vi "Initalize SR830(SubVI).vi"(0 "簇":T1={"initialize"=enum."SR830", "6221"={"6221 Resource"="GPIB0::24::INSTR", "Delta status"=FALSE, "电流|RMS(A)"=0.0}, "SR830+6221"={"source"=0, "Current(A)"=0.0, "阻抗(Ohm)"=0.0, "SR830 1"=FALSE, "SR830 2"=FALSE, "SR830 3"=FALSE, "SR830 4"=FALSE, "VISA 1"="", "VISA 2"="", "VISA 3"="", "VISA 4"="", "Reserve 1"=0, "Reserve 2"=-1, "Reserve 3"=-1, "Reserve 4"=-1, "Sensitivity 1"=-1, "Sensitivity 2"=0, "Sensitivity 3"=-1, "Sensitivity 4"=-1, "量程入 1"=0, "量程入 2"=0, "量程入 3"=0, "量程入 4"=0}, "2400"={"2400"=FALSE, "VISA"="", "Output Level (0)"=1e-05, "Compliance  Level (0.1)"=10.0}, "ch"={"ch"=[], "current"=[], "change?"=[], "holding current\nwhen change ch?"=FALSE}, "Instrument"={"325 Resource "="GPIB0::13::INSTR", "Input (0:A) 325"=0, "Heater Output (1:1) 325"=1, "340 Resource"="GPIB0::14::INSTR", "Input (0:A) 340"=0, "Loop (0: 1)"=0, "Input (0:B) 340"=1, "Loop (1: 1)"=0, "340 Status"=refnum, "Instrument Type"=enum."PPMS-Rotate", "quantum design"=refnum, "semaphore 325"=refnum, "TCP master instance"=refnum, "M24C Resource"="GPIB0::24::INSTR", "4G supply"="GPIB0::24::INSTR", "Temp Status 24C"=refnum, "Temp"=refnum, "9T信号"=refnum, "limit"={"Field limit"=0.0, "Field rate limit"=0.0, "Temp limit"=0.0, "Temp low limit"=0.0, "Temp rate limit "=0.0}, "4g supply status"=refnum, "vi路径"="", "in-plane"="", "out-plane"="", "in-plane signal"=FALSE, "out-plane signal"=FALSE, "in plane 信号"=refnum, "pzt volt"=refnum, "Aborting"=refnum, "数据文件"=refnum, "warning"=refnum, "750 visa"="", "750 rotate"="", "335 Status 2"=refnum, "335 Resource "="GPIB0::24::INSTR", "Input (0:A) 335"=0, "Input (0:B) 335"=1, "Heater Output (1:1) 335"=1, "semaphore 340"=refnum, "semaphore 335"=refnum, "325 Status"=refnum, "semaphore 750"=refnum, "750 field status"=refnum, "camg 振荡状态"=refnum, "列表框"=refnum, "编辑列表框？"=refnum, "camg Rate"=refnum, "行数"=refnum}, "2614B"={"2614B chA"=FALSE, "2614B chB"=FALSE, "VISA"=""}, "33522b"={"33522b resource name"="GPIB0::16::INSTR", "零电压"=0.0, "最大电压"=148.0, "间隔"=4.0, "最小电压"=-48.0, "PZT Scan?"=FALSE}, "gating type"=enum."2614(daul)", "层数"=0, "行数"=0, "是否处理"=[]} {"Instrument"."Loop (1: 1)" items=["1"=1, "2"=2]; "Instrument"."Loop (0: 1)" items=["1"=1, "2"=2]; "Instrument"."Input (0:B) 340" items=["A", "B", "C", "D"]; "Instrument"."Heater Output (1:1) 335" items=["1"=1, "2"=2]; "Instrument"."Input (0:B) 335" items=["A", "B"]; "Instrument"."Input (0:A) 335" items=["A", "B"]; "Instrument"."Heater Output (1:1) 325" items=["1"=1, "2"=2]; "Instrument"."Input (0:A) 325" items=["A", "B"]; "Instrument"."Input (0:A) 340" items=["1"=1, "2"=2]; "SR830+6221"."Sensitivity 4" items=["Auto Gain"=-1, "2 nV/fA"=0, "5 nV/fA"=1, "10 nV/fA"=2, "20 nV/fA"=3, "50 nV/fA"=4, "100 nV/fA"=5, "200 nV/fA"=6, "500 nV/fA"=7, "1 uV/pA"=8, "2 uV/pA"=9, "5 uV/pA"=10, "10 uV/pA"=11, "20 uV/pA"=12, "50 uV/pA"=13, "100 uV/pA"=14, "200 uV/pA"=15, "500 uV/pA"=16, "1 mV/nA"=17, "2 mV/nA"=18, "5 mV/nA"=19, "10 mV/nA"=20, "20 mV/nA"=21, "50 mV/nA"=22, "100 mV/nA"=23, "200 mV/nA"=24, "500 mV/mA"=25, "1 V/uA"=26]; "SR830+6221"."Sensitivity 3" items=["Auto Gain"=-1, "2 nV/fA"=0, "5 nV/fA"=1, "10 nV/fA"=2, "20 nV/fA"=3, "50 nV/fA"=4, "100 nV/fA"=5, "200 nV/fA"=6, "500 nV/fA"=7, "1 uV/pA"=8, "2 uV/pA"=9, "5 uV/pA"=10, "10 uV/pA"=11, "20 uV/pA"=12, "50 uV/pA"=13, "100 uV/pA"=14, "200 uV/pA"=15, "500 uV/pA"=16, "1 mV/nA"=17, "2 mV/nA"=18, "5 mV/nA"=19, "10 mV/nA"=20, "20 mV/nA"=21, "50 mV/nA"=22, "100 mV/nA"=23, "200 mV/nA"=24, "500 mV/mA"=25, "1 V/uA"=26]; "SR830+6221"."Sensitivity 1" items=["Auto Gain"=-1, "2 nV/fA"=0, "5 nV/fA"=1, "10 nV/fA"=2, "20 nV/fA"=3, "50 nV/fA"=4, "100 nV/fA"=5, "200 nV/fA"=6, "500 nV/fA"=7, "1 uV/pA"=8, "2 uV/pA"=9, "5 uV/pA"=10, "10 uV/pA"=11, "20 uV/pA"=12, "50 uV/pA"=13, "100 uV/pA"=14, "200 uV/pA"=15, "500 uV/pA"=16, "1 mV/nA"=17, "2 mV/nA"=18, "5 mV/nA"=19, "10 mV/nA"=20, "20 mV/nA"=21, "50 mV/nA"=22, "100 mV/nA"=23, "200 mV/nA"=24, "500 mV/mA"=25, "1 V/uA"=26]; "SR830+6221"."Sensitivity 2" items=["Auto Gain"=-1, "2 nV/fA"=0, "5 nV/fA"=1, "10 nV/fA"=2, "20 nV/fA"=3, "50 nV/fA"=4, "100 nV/fA"=5, "200 nV/fA"=6, "500 nV/fA"=7, "1 uV/pA"=8, "2 uV/pA"=9, "5 uV/pA"=10, "10 uV/pA"=11, "20 uV/pA"=12, "50 uV/pA"=13, "100 uV/pA"=14, "200 uV/pA"=15, "500 uV/pA"=16, "1 mV/nA"=17, "2 mV/nA"=18, "5 mV/nA"=19, "10 mV/nA"=20, "20 mV/nA"=21, "50 mV/nA"=22, "100 mV/nA"=23, "200 mV/nA"=24, "500 mV/mA"=25, "1 V/uA"=26]; "SR830+6221"."Reserve 4" items=["Auto Gain"=-1, "2 nV/fA"=0, "5 nV/fA"=1, "10 nV/fA"=2, "20 nV/fA"=3, "50 nV/fA"=4, "100 nV/fA"=5, "200 nV/fA"=6, "500 nV/fA"=7, "1 uV/pA"=8, "2 uV/pA"=9, "5 uV/pA"=10, "10 uV/pA"=11, "20 uV/pA"=12, "50 uV/pA"=13, "100 uV/pA"=14, "200 uV/pA"=15, "500 uV/pA"=16, "1 mV/nA"=17, "2 mV/nA"=18, "5 mV/nA"=19, "10 mV/nA"=20, "20 mV/nA"=21, "50 mV/nA"=22, "100 mV/nA"=23, "200 mV/nA"=24, "500 mV/mA"=25, "1 V/uA"=26]; "SR830+6221"."Reserve 3" items=["Auto Reserve"=-1, "High Reserve"=0, "Normal"=1, "Low Noise"=2]; "SR830+6221"."Reserve 2" items=["Auto Reserve"=-1, "High Reserve"=0, "Normal"=1, "Low Noise"=2]; "SR830+6221"."Reserve 1" items=["Auto Reserve"=-1, "High Reserve"=0, "Normal"=1, "Low Noise"=2]; "SR830+6221"."source" items=["SR830 1", "SR830 2", "SR830 3", "SR830 4"]}, 9 "字符串":string) -> (4 "输出簇":T1={"initialize"=enum."SR830", "6221"={"6221 Resource"="GPIB0::24::INSTR", "Delta status"=FALSE, "电流|RMS(A)"=0.0}, "SR830+6221"={"source"=0, "Current(A)"=0.0, "阻抗(Ohm)"=0.0, "SR830 1"=FALSE, "SR830 2"=FALSE, "SR830 3"=FALSE, "SR830 4"=FALSE, "VISA 1"="", "VISA 2"="", "VISA 3"="", "VISA 4"="", "Reserve 1"=0, "Reserve 2"=-1, "Reserve 3"=-1, "Reserve 4"=-1, "Sensitivity 1"=-1, "Sensitivity 2"=0, "Sensitivity 3"=-1, "Sensitivity 4"=-1, "量程入 1"=0, "量程入 2"=0, "量程入 3"=0, "量程入 4"=0}, "2400"={"2400"=FALSE, "VISA"="", "Output Level (0)"=1e-05, "Compliance  Level (0.1)"=10.0}, "ch"={"ch"=[], "current"=[], "change?"=[], "holding current\nwhen change ch?"=FALSE}, "Instrument"={"325 Resource "="GPIB0::13::INSTR", "Input (0:A) 325"=0, "Heater Output (1:1) 325"=1, "340 Resource"="GPIB0::14::INSTR", "Input (0:A) 340"=0, "Loop (0: 1)"=0, "Input (0:B) 340"=1, "Loop (1: 1)"=0, "340 Status"=refnum, "Instrument Type"=enum."PPMS-Rotate", "quantum design"=refnum, "semaphore 325"=refnum, "TCP master instance"=refnum, "M24C Resource"="GPIB0::24::INSTR", "4G supply"="GPIB0::24::INSTR", "Temp Status 24C"=refnum, "Temp"=refnum, "9T信号"=refnum, "limit"={"Field limit"=0.0, "Field rate limit"=0.0, "Temp limit"=0.0, "Temp low limit"=0.0, "Temp rate limit "=0.0}, "4g supply status"=refnum, "vi路径"="", "in-plane"="", "out-plane"="", "in-plane signal"=FALSE, "out-plane signal"=FALSE, "in plane 信号"=refnum, "pzt volt"=refnum, "Aborting"=refnum, "数据文件"=refnum, "warning"=refnum, "750 visa"="", "750 rotate"="", "335 Status 2"=refnum, "335 Resource "="GPIB0::24::INSTR", "Input (0:A) 335"=0, "Input (0:B) 335"=1, "Heater Output (1:1) 335"=1, "semaphore 340"=refnum, "semaphore 335"=refnum, "325 Status"=refnum, "semaphore 750"=refnum, "750 field status"=refnum, "camg 振荡状态"=refnum, "列表框"=refnum, "编辑列表框？"=refnum, "camg Rate"=refnum, "行数"=refnum}, "2614B"={"2614B chA"=FALSE, "2614B chB"=FALSE, "VISA"=""}, "33522b"={"33522b resource name"="GPIB0::16::INSTR", "零电压"=0.0, "最大电压"=148.0, "间隔"=4.0, "最小电压"=-48.0, "PZT Scan?"=FALSE}, "gating type"=enum."2614(daul)", "层数"=0, "行数"=0, "是否处理"=[]} {"Instrument"."Loop (1: 1)" items=["1"=1, "2"=2]; "Instrument"."Loop (0: 1)" items=["1"=1, "2"=2]; "Instrument"."Input (0:B) 340" items=["A", "B", "C", "D"]; "Instrument"."Heater Output (1:1) 335" items=["1"=1, "2"=2]; "Instrument"."Input (0:B) 335" items=["A", "B"]; "Instrument"."Input (0:A) 335" items=["A", "B"]; "Instrument"."Heater Output (1:1) 325" items=["1"=1, "2"=2]; "Instrument"."Input (0:A) 325" items=["A", "B"]; "Instrument"."Input (0:A) 340" items=["1"=1, "2"=2]; "SR830+6221"."Sensitivity 4" items=["Auto Gain"=-1, "2 nV/fA"=0, "5 nV/fA"=1, "10 nV/fA"=2, "20 nV/fA"=3, "50 nV/fA"=4, "100 nV/fA"=5, "200 nV/fA"=6, "500 nV/fA"=7, "1 uV/pA"=8, "2 uV/pA"=9, "5 uV/pA"=10, "10 uV/pA"=11, "20 uV/pA"=12, "50 uV/pA"=13, "100 uV/pA"=14, "200 uV/pA"=15, "500 uV/pA"=16, "1 mV/nA"=17, "2 mV/nA"=18, "5 mV/nA"=19, "10 mV/nA"=20, "20 mV/nA"=21, "50 mV/nA"=22, "100 mV/nA"=23, "200 mV/nA"=24, "500 mV/mA"=25, "1 V/uA"=26]; "SR830+6221"."Sensitivity 3" items=["Auto Gain"=-1, "2 nV/fA"=0, "5 nV/fA"=1, "10 nV/fA"=2, "20 nV/fA"=3, "50 nV/fA"=4, "100 nV/fA"=5, "200 nV/fA"=6, "500 nV/fA"=7, "1 uV/pA"=8, "2 uV/pA"=9, "5 uV/pA"=10, "10 uV/pA"=11, "20 uV/pA"=12, "50 uV/pA"=13, "100 uV/pA"=14, "200 uV/pA"=15, "500 uV/pA"=16, "1 mV/nA"=17, "2 mV/nA"=18, "5 mV/nA"=19, "10 mV/nA"=20, "20 mV/nA"=21, "50 mV/nA"=22, "100 mV/nA"=23, "200 mV/nA"=24, "500 mV/mA"=25, "1 V/uA"=26]; "SR830+6221"."Sensitivity 1" items=["Auto Gain"=-1, "2 nV/fA"=0, "5 nV/fA"=1, "10 nV/fA"=2, "20 nV/fA"=3, "50 nV/fA"=4, "100 nV/fA"=5, "200 nV/fA"=6, "500 nV/fA"=7, "1 uV/pA"=8, "2 uV/pA"=9, "5 uV/pA"=10, "10 uV/pA"=11, "20 uV/pA"=12, "50 uV/pA"=13, "100 uV/pA"=14, "200 uV/pA"=15, "500 uV/pA"=16, "1 mV/nA"=17, "2 mV/nA"=18, "5 mV/nA"=19, "10 mV/nA"=20, "20 mV/nA"=21, "50 mV/nA"=22, "100 mV/nA"=23, "200 mV/nA"=24, "500 mV/mA"=25, "1 V/uA"=26]; "SR830+6221"."Sensitivity 2" items=["Auto Gain"=-1, "2 nV/fA"=0, "5 nV/fA"=1, "10 nV/fA"=2, "20 nV/fA"=3, "50 nV/fA"=4, "100 nV/fA"=5, "200 nV/fA"=6, "500 nV/fA"=7, "1 uV/pA"=8, "2 uV/pA"=9, "5 uV/pA"=10, "10 uV/pA"=11, "20 uV/pA"=12, "50 uV/pA"=13, "100 uV/pA"=14, "200 uV/pA"=15, "500 uV/pA"=16, "1 mV/nA"=17, "2 mV/nA"=18, "5 mV/nA"=19, "10 mV/nA"=20, "20 mV/nA"=21, "50 mV/nA"=22, "100 mV/nA"=23, "200 mV/nA"=24, "500 mV/mA"=25, "1 V/uA"=26]; "SR830+6221"."Reserve 4" items=["Auto Gain"=-1, "2 nV/fA"=0, "5 nV/fA"=1, "10 nV/fA"=2, "20 nV/fA"=3, "50 nV/fA"=4, "100 nV/fA"=5, "200 nV/fA"=6, "500 nV/fA"=7, "1 uV/pA"=8, "2 uV/pA"=9, "5 uV/pA"=10, "10 uV/pA"=11, "20 uV/pA"=12, "50 uV/pA"=13, "100 uV/pA"=14, "200 uV/pA"=15, "500 uV/pA"=16, "1 mV/nA"=17, "2 mV/nA"=18, "5 mV/nA"=19, "10 mV/nA"=20, "20 mV/nA"=21, "50 mV/nA"=22, "100 mV/nA"=23, "200 mV/nA"=24, "500 mV/mA"=25, "1 V/uA"=26]; "SR830+6221"."Reserve 3" items=["Auto Reserve"=-1, "High Reserve"=0, "Normal"=1, "Low Noise"=2]; "SR830+6221"."Reserve 2" items=["Auto Reserve"=-1, "High Reserve"=0, "Normal"=1, "Low Noise"=2]; "SR830+6221"."Reserve 1" items=["Auto Reserve"=-1, "High Reserve"=0, "Normal"=1, "Low Noise"=2]; "SR830+6221"."source" items=["SR830 1", "SR830 2", "SR830 3", "SR830 4"]})   [LabVIEW 2019, in "initialize.lvlib"]
uses:
  initialize.lvlib
  lib/Keithley 622x/Configure/6221 Wave/Typedefs/KE6221 -- Wave Sine Wave Params.ctl
  lib/Keithley 622x/Configure/6221 Wave/Low Level/Typedefs/KE6221 -- Wave Frequency.ctl
  lib/Keithley 622x/Configure/6221 Wave/Low Level/Typedefs/KE6221 -- Wave Amplitude.ctl
  lib/Keithley 622x/Configure/Source/Typedefs/KE622x -- Current Level.ctl
  lib/Keithley 622x/Configure/6221 Wave/Low Level/Typedefs/KE6221 -- Wave Ranging Mode.ctl
  lib/Keithley 622x/Configure/Source/Typedefs/KE622x -- Current Ranges.ctl
  lib/Keithley 622x/Configure/6221 Wave/Low Level/Typedefs/KE6221 -- Wave Playback Mode.ctl
  lib/Keithley 622x/Configure/6221 Wave/Low Level/Typedefs/KE6221 -- Wave Playback Time.ctl
  lib/Keithley 622x/Configure/6221 Wave/Low Level/Typedefs/KE6221 -- Wave Playback Num Cycles.ctl
  lib/Keithley 622x/Configure/6221 Wave/Low Level/Typedefs/KE6221 -- Wave Phase Marker.ctl
  lib/Keithley 622x/Configure/Trigger/Low Level/Typedefs/KE622x -- Trig Link Line.ctl
  ctl/config.ctl
  <vilib>/NI/Modbus Library/API/Master/Modbus Master.lvclass
  ctl/initialize.ctl
  ctl/Instrument.ctl
  ctl/335 state.ctl
  ctl/Instrument Type.ctl
  lib/QDInstrument.dll
  ctl/limit.ctl
  ctl/9T mag field stauts.ctl
  ctl/warning.ctl
  ctl/Gating type.ctl
  lib/Keithley 622x/Configure/6221 Wave/Low Level/Typedefs/KE6221 -- Wave Type.ctl
  lib/Keithley 622x/Keithley 622x.lvlib
  SubVI.lvlib
  User lib.lvlib
panel:
  in  "同步 3":bool
  in  "同步 2":bool
  in  "同步":bool
  in  "6221(SR830做源可忽略）":T19={"Sine Wave Params In"={"Frequency (Hz)"=1000.0, "Amplitude (A)"=0.001, "Offset (A)"=0.0, "Ranging Mode"=enum."Best", "Fixed Range"=enum."2mA", "Playback Mode"=enum."Time", "Time (s)"=999999.999, "Num Cycles"=1.0, "Phase\nMarker?"=TRUE, "Phase Marker (deg)"=0.0, "Trig Link Line"=enum."3"}, "RMS Amplitude (A)"=0.001} {"RMS Amplitude (A)" min=2e-12 max=0.105 format="%.3p"; "Sine Wave Params In"."Offset (A)" min=-0.105 max=0.105 format="%.4p"; "Sine Wave Params In"."Num Cycles" min=0.001 max=99999999900.0 format="%.3p"; "Sine Wave Params In"."Time (s)" min=1e-07 max=999999.999 format="%.3p"; "Sine Wave Params In"."Phase Marker (deg)" min=0.0 max=360.0 format="%.3f"; "Sine Wave Params In"."Amplitude (A)" min=2e-12 max=0.105 format="%.3p"; "Sine Wave Params In"."Frequency (Hz)" min=0.001 max=100000.0 format="%.3p"}
  in  "仪器设置":T20={"ID Query"=FALSE, "Reset"=FALSE, "Sensitivity 2"=-1, "Sensitivity 1"=-1, "SR830源配合的阻抗（6221做源可忽略）"=0.0, "SR830 2"=FALSE, "SR830 3"=FALSE, "SR830 4"=FALSE, "Sensitivity 3"=-1, "Sensitivity 4"=-1, "source"=0, "SR830 1"=FALSE, "Reserve 1"=-1, "Reserve 2"=-1, "Reserve 3"=-1, "Reserve 4"=-1} {"Reserve 4" items=["Auto Reserve"=-1, "High Reserve"=0, "Normal"=1, "Low Noise"=2]; "Reserve 3" items=["Auto Reserve"=-1, "High Reserve"=0, "Normal"=1, "Low Noise"=2]; "Reserve 2" items=["Auto Reserve"=-1, "High Reserve"=0, "Normal"=1, "Low Noise"=2]; "Reserve 1" items=["Auto Reserve"=-1, "High Reserve"=0, "Normal"=1, "Low Noise"=2]; "source" items=["SR830 1", "SR830 2", "SR830 3", "SR830 4", "6221"]; "Sensitivity 4" items=["Auto Gain"=-1, "2 nV/fA"=0, "5 nV/fA"=1, "10 nV/fA"=2, "20 nV/fA"=3, "50 nV/fA"=4, "100 nV/fA"=5, "200 nV/fA"=6, "500 nV/fA"=7, "1 uV/pA"=8, "2 uV/pA"=9, "5 uV/pA"=10, "10 uV/pA"=11, "20 uV/pA"=12, "50 uV/pA"=13, "100 uV/pA"=14, "200 uV/pA"=15, "500 uV/pA"=16, "1 mV/nA"=17, "2 mV/nA"=18, "5 mV/nA"=19, "10 mV/nA"=20, "20 mV/nA"=21, "50 mV/nA"=22, "100 mV/nA"=23, "200 mV/nA"=24, "500 mV/mA"=25, "1 V/uA"=26]; "Sensitivity 3" items=["Auto Gain"=-1, "2 nV/fA"=0, "5 nV/fA"=1, "10 nV/fA"=2, "20 nV/fA"=3, "50 nV/fA"=4, "100 nV/fA"=5, "200 nV/fA"=6, "500 nV/fA"=7, "1 uV/pA"=8, "2 uV/pA"=9, "5 uV/pA"=10, "10 uV/pA"=11, "20 uV/pA"=12, "50 uV/pA"=13, "100 uV/pA"=14, "200 uV/pA"=15, "500 uV/pA"=16, "1 mV/nA"=17, "2 mV/nA"=18, "5 mV/nA"=19, "10 mV/nA"=20, "20 mV/nA"=21, "50 mV/nA"=22, "100 mV/nA"=23, "200 mV/nA"=24, "500 mV/mA"=25, "1 V/uA"=26]; "Sensitivity 1" items=["Auto Gain"=-1, "2 nV/fA"=0, "5 nV/fA"=1, "10 nV/fA"=2, "20 nV/fA"=3, "50 nV/fA"=4, "100 nV/fA"=5, "200 nV/fA"=6, "500 nV/fA"=7, "1 uV/pA"=8, "2 uV/pA"=9, "5 uV/pA"=10, "10 uV/pA"=11, "20 uV/pA"=12, "50 uV/pA"=13, "100 uV/pA"=14, "200 uV/pA"=15, "500 uV/pA"=16, "1 mV/nA"=17, "2 mV/nA"=18, "5 mV/nA"=19, "10 mV/nA"=20, "20 mV/nA"=21, "50 mV/nA"=22, "100 mV/nA"=23, "200 mV/nA"=24, "500 mV/mA"=25, "1 V/uA"=26]; "Sensitivity 2" items=["Auto Gain"=-1, "2 nV/fA"=0, "5 nV/fA"=1, "10 nV/fA"=2, "20 nV/fA"=3, "50 nV/fA"=4, "100 nV/fA"=5, "200 nV/fA"=6, "500 nV/fA"=7, "1 uV/pA"=8, "2 uV/pA"=9, "5 uV/pA"=10, "10 uV/pA"=11, "20 uV/pA"=12, "50 uV/pA"=13, "100 uV/pA"=14, "200 uV/pA"=15, "500 uV/pA"=16, "1 mV/nA"=17, "2 mV/nA"=18, "5 mV/nA"=19, "10 mV/nA"=20, "20 mV/nA"=21, "50 mV/nA"=22, "100 mV/nA"=23, "200 mV/nA"=24, "500 mV/mA"=25, "1 V/uA"=26]}
  in  "滤波设置 4":T21={"Time Constant "=8, "Low Pass Filter Slope "=1, "Enable Sync Filter "=TRUE} {"Low Pass Filter Slope" items=["6 dB/oct", "12 dB/oct", "18 db/oct", "24 dB/oct"]; "Time Constant" items=["10 us", "30 us", "100 us", "300 us", "1 ms", "3 ms", "10 ms", "30 ms", "100 ms", "300 ms", "1 s", "3 s", "10 s", "30 s", "100 s", "300 s", "1 ks", "3 ks", "10 ks", "30 ks"]}
  in  "滤波设置 3":T21={"Time Constant "=8, "Low Pass Filter Slope "=1, "Enable Sync Filter "=TRUE} {"Low Pass Filter Slope" items=["6 dB/oct", "12 dB/oct", "18 db/oct", "24 dB/oct"]; "Time Constant" items=["10 us", "30 us", "100 us", "300 us", "1 ms", "3 ms", "10 ms", "30 ms", "100 ms", "300 ms", "1 s", "3 s", "10 s", "30 s", "100 s", "300 s", "1 ks", "3 ks", "10 ks", "30 ks"]}
  in  "滤波设置 2":T21={"Time Constant "=8, "Low Pass Filter Slope "=1, "Enable Sync Filter "=TRUE} {"Low Pass Filter Slope" items=["6 dB/oct", "12 dB/oct", "18 db/oct", "24 dB/oct"]; "Time Constant" items=["10 us", "30 us", "100 us", "300 us", "1 ms", "3 ms", "10 ms", "30 ms", "100 ms", "300 ms", "1 s", "3 s", "10 s", "30 s", "100 s", "300 s", "1 ks", "3 ks", "10 ks", "30 ks"]}
  in  "参考信号 4":T22={"Reference Source"=1, "External Reference Trigger  "=0, "Detection Harmonic Number "=1.0, "Manual Phase (Degree)"=0.0, "Auto Phase "=FALSE, "Sine Output Amplitude (V)"=1.0, "Internal Reference Frequency (Hz)"=13.0} {"External Reference Trigger" items=["Sine Zero Crossing", "TTL Rising Edge", "TTL Falling Edge"]; "Reference Source" items=["External", "Internal"]}
  in  "参考信号 3":T22={"Reference Source"=1, "External Reference Trigger  "=0, "Detection Harmonic Number "=1.0, "Manual Phase (Degree)"=0.0, "Auto Phase "=FALSE, "Sine Output Amplitude (V)"=1.0, "Internal Reference Frequency (Hz)"=13.0} {"External Reference Trigger" items=["Sine Zero Crossing", "TTL Rising Edge", "TTL Falling Edge"]; "Reference Source" items=["External", "Internal"]}
  in  "参考信号 2":T22={"Reference Source"=1, "External Reference Trigger  "=0, "Detection Harmonic Number "=1.0, "Manual Phase (Degree)"=0.0, "Auto Phase "=FALSE, "Sine Output Amplitude (V)"=1.0, "Internal Reference Frequency (Hz)"=13.0} {"External Reference Trigger" items=["Sine Zero Crossing", "TTL Rising Edge", "TTL Falling Edge"]; "Reference Source" items=["External", "Internal"]}
  in  "输入信号 4":T23={"Input Notch Filter "=0, "Input Shield Grounding"=0, "Input Coupling "=0, "Input Connection  "=1} {"Input Connection" items=["Single-Ended Voltage", "Differential Voltage", "1 MOhm Current Gain", "100 MOhm Current Gain"]; "Input Coupling" items=["AC", "DC"]; "Input Shield Grounding" items=["Float", "Ground"]; "Input Notch Filter" items=["None", "Line Notch", "2x Line Notch", "Both Notch Filters"]}
  in  "输入信号 3":T23={"Input Notch Filter "=0, "Input Shield Grounding"=0, "Input Coupling "=0, "Input Connection  "=1} {"Input Connection" items=["Single-Ended Voltage", "Differential Voltage", "1 MOhm Current Gain", "100 MOhm Current Gain"]; "Input Coupling" items=["AC", "DC"]; "Input Shield Grounding" items=["Float", "Ground"]; "Input Notch Filter" items=["None", "Line Notch", "2x Line Notch", "Both Notch Filters"]}
  in  "输入信号 2":T23={"Input Notch Filter "=0, "Input Shield Grounding"=0, "Input Coupling "=0, "Input Connection  "=1} {"Input Connection" items=["Single-Ended Voltage", "Differential Voltage", "1 MOhm Current Gain", "100 MOhm Current Gain"]; "Input Coupling" items=["AC", "DC"]; "Input Shield Grounding" items=["Float", "Ground"]; "Input Notch Filter" items=["None", "Line Notch", "2x Line Notch", "Both Notch Filters"]}
  in  "滤波设置":T21={"Time Constant "=8, "Low Pass Filter Slope "=1, "Enable Sync Filter "=TRUE} {"Low Pass Filter Slope" items=["6 dB/oct", "12 dB/oct", "18 db/oct", "24 dB/oct"]; "Time Constant" items=["10 us", "30 us", "100 us", "300 us", "1 ms", "3 ms", "10 ms", "30 ms", "100 ms", "300 ms", "1 s", "3 s", "10 s", "30 s", "100 s", "300 s", "1 ks", "3 ks", "10 ks", "30 ks"]}
  in  "参考信号":T22={"Reference Source"=1, "External Reference Trigger  "=0, "Detection Harmonic Number "=1.0, "Manual Phase (Degree)"=0.0, "Auto Phase "=FALSE, "Sine Output Amplitude (V)"=1.0, "Internal Reference Frequency (Hz)"=13.0} {"External Reference Trigger" items=["Sine Zero Crossing", "TTL Rising Edge", "TTL Falling Edge"]; "Reference Source" items=["External", "Internal"]}
  in  "输入信号":T23={"Input Notch Filter "=0, "Input Shield Grounding"=0, "Input Coupling "=0, "Input Connection  "=1} {"Input Connection" items=["Single-Ended Voltage", "Differential Voltage", "1 MOhm Current Gain", "100 MOhm Current Gain"]; "Input Coupling" items=["AC", "DC"]; "Input Shield Grounding" items=["Float", "Ground"]; "Input Notch Filter" items=["None", "Line Notch", "2x Line Notch", "Both Notch Filters"]}
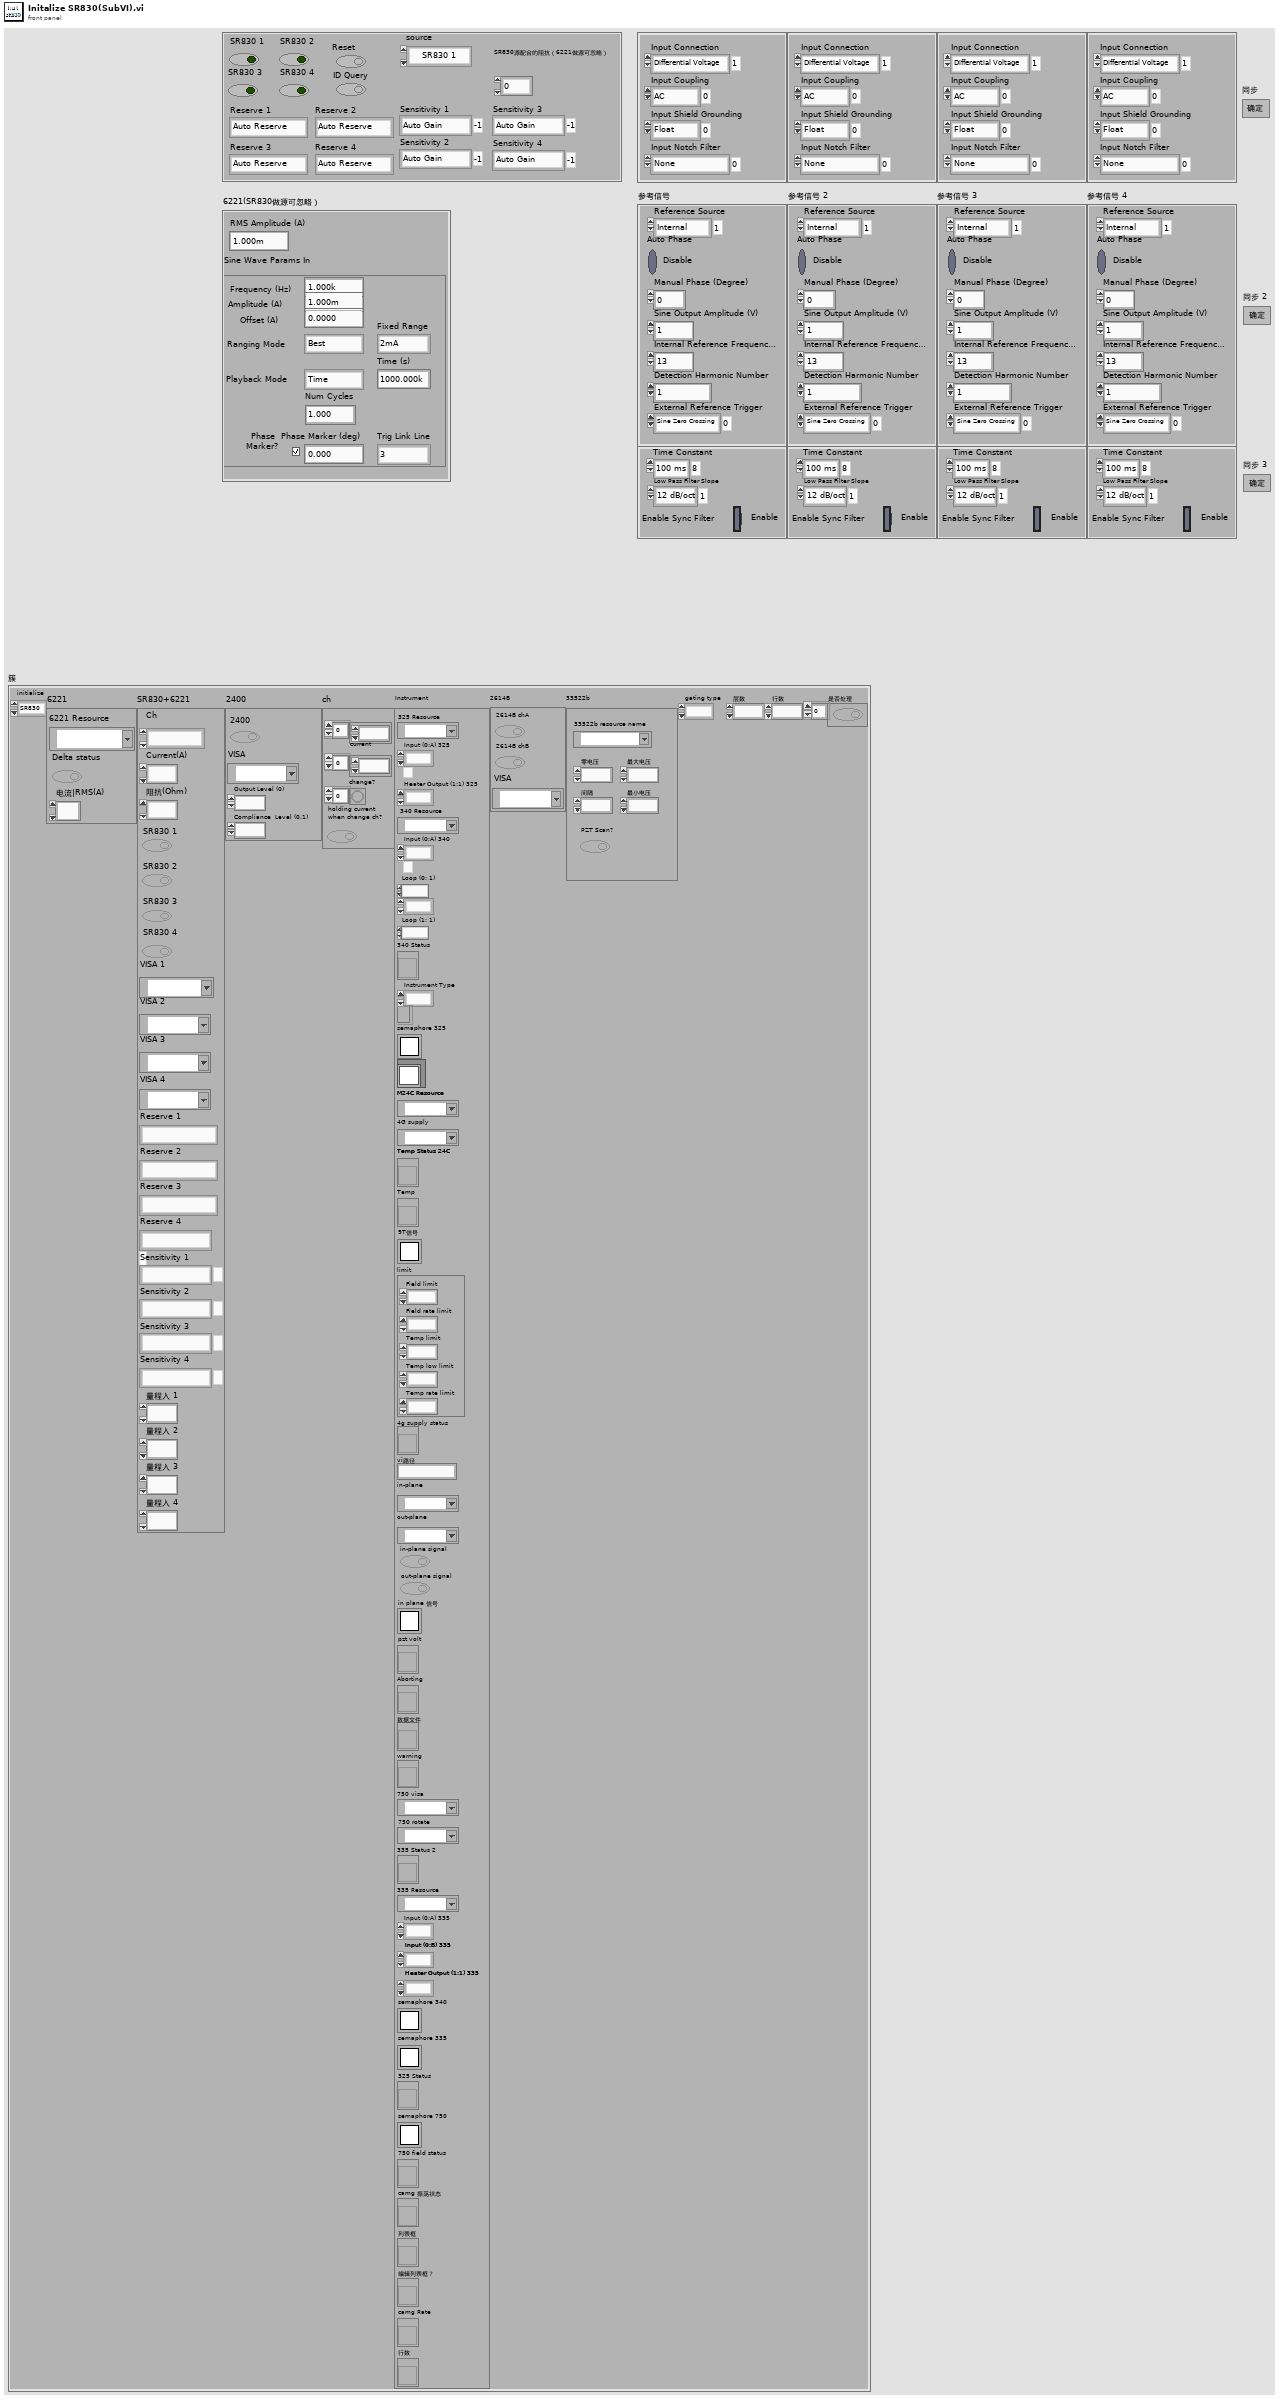
[diagram p1: front panel]
types:
  T1 = typedef "config.ctl" = cluster{"initialize":T2, "6221":cluster{"6221 Resource":refnum<visa-resource-name>, "Delta status":bool, "电流|RMS(A)":dbl}, "SR830+6221":cluster{"source":u16, "Current(A)":dbl, "阻抗(Ohm)":dbl, "SR830 1":bool, "SR830 2":bool, "SR830 3":bool, "SR830 4":bool, "VISA 1":refnum<visa-resource-name>, "VISA 2":refnum<visa-resource-name>, "VISA 3":refnum<visa-resource-name>, "VISA 4":refnum<visa-resource-name>, "Reserve 1":i16, "Reserve 2":i16, "Reserve 3":i16, "Reserve 4":i16, "Sensitivity 1":i16, "Sensitivity 2":i16, "Sensitivity 3":i16, "Sensitivity 4":i16, "量程入 1":i32, "量程入 2":i32, "量程入 3":i32, "量程入 4":i32}, "2400":cluster{"2400":bool, "VISA":refnum<visa-resource-name>, "Output Level (0)":dbl, "Compliance  Level (0.1)":dbl}, "ch":cluster{"ch":i32[], "current":dbl[], "change?":bool[], "holding current\nwhen change ch?":bool}, "Instrument":T3, "2614B":cluster{"2614B chA":bool, "2614B chB":bool, "VISA":refnum<visa-resource-name>}, "33522b":cluster{"33522b resource name":refnum<visa-resource-name>, "零电压":dbl, "最大电压":dbl, "间隔":dbl, "最小电压":dbl, "PZT Scan?":bool}, "gating type":T7, "层数":i32, "行数":i32, "是否处理":bool[]}
  T2 = typedef "initialize.ctl" = enum16{"SR830", "keithley6221-SR830", "Delta", "Delta-tunnelling", "keithley6221-2182-DC", "PZT", "4200"}
  T3 = typedef "Instrument.ctl" = cluster{"325 Resource ":refnum<visa-resource-name>, "Input (0:A) 325":u16, "Heater Output (1:1) 325":u16, "340 Resource":refnum<visa-resource-name>, "Input (0:A) 340":u16, "Loop (0: 1)":u16, "Input (0:B) 340":u16, "Loop (1: 1)":u16, "340 Status":refnum<vi>, "Instrument Type":T4, "quantum design":refnum<k24>, "semaphore 325":T5, "TCP master instance":refnum<class "Modbus Master.lvclass">, "M24C Resource":refnum<visa-resource-name>, "4G supply":refnum<visa-resource-name>, "Temp Status 24C":refnum<vi>, "Temp":refnum<vi>, "9T信号":T5, "limit":T6, "4g supply status":refnum<vi>, "vi路径":string, "in-plane":refnum<visa-resource-name>, "out-plane":refnum<visa-resource-name>, "in-plane signal":bool, "out-plane signal":bool, "in plane 信号":T5, "pzt volt":refnum<vi>, "Aborting":refnum<vi>, "数据文件":refnum<vi>, "warning":refnum<vi>, "750 visa":refnum<visa-resource-name>, "750 rotate":refnum<visa-resource-name>, "335 Status 2":refnum<vi>, "335 Resource ":refnum<visa-resource-name>, "Input (0:A) 335":u16, "Input (0:B) 335":u16, "Heater Output (1:1) 335":u16, "semaphore 340":T5, "semaphore 335":T5, "325 Status":refnum<vi>, "semaphore 750":T5, "750 field status":refnum<vi>, "camg 振荡状态":refnum<vi>, "列表框":refnum<vi>, "编辑列表框？":refnum<vi>, "camg Rate":refnum<vi>, "行数":refnum<vi>}
  T4 = typedef "Instrument Type.ctl" = enum16{"PPMS", "VersaLab", "DynaCool", "SVSM", "PPMS-Rotate", "Lakeshore335", "lengtou2", "9T mag", "9T cmag rotate", "test"}
  T5 = typedef "Semaphore RefNum" = refnum<k1>
  T6 = typedef "limit.ctl" = cluster{"Field limit":dbl, "Field rate limit":dbl, "Temp limit":dbl, "Temp low limit":dbl, "Temp rate limit ":dbl}
  T7 = typedef "Gating type.ctl" = enum32{"null", "2614(daul)", "2400"}
  T8 = typedef "Keithley 622x.lvlib/KE6221 -- Wave Sine Wave Params.ctl" = cluster{"Frequency (Hz)":T9, "Amplitude (A)":T10, "Offset (A)":T11, "Ranging Mode":T12, "Fixed Range":T13, "Playback Mode":T14, "Time (s)":T15, "Num Cycles":T16, "Phase\nMarker?":bool, "Phase Marker (deg)":T17, "Trig Link Line":T18}
  T9 = typedef "Keithley 622x.lvlib/KE6221 -- Wave Frequency.ctl" = dbl
  T10 = typedef "Keithley 622x.lvlib/KE6221 -- Wave Amplitude.ctl" = dbl
  T11 = typedef "Keithley 622x.lvlib/KE622x -- Current Level.ctl" = dbl
  T12 = typedef "Keithley 622x.lvlib/KE6221 -- Wave Ranging Mode.ctl" = enum16{"Best", "Fixed"}
  T13 = typedef "Keithley 622x.lvlib/KE622x -- Current Ranges.ctl" = enum16{"2nA", "20nA", "200nA", "2uA", "20uA", "200uA", "2mA", "20mA", "100mA"}
  T14 = typedef "Keithley 622x.lvlib/KE6221 -- Wave Playback Mode.ctl" = enum16{"Time", "Num Cycles"}
  T15 = typedef "Keithley 622x.lvlib/KE6221 -- Wave Playback Time.ctl" = dbl
  T16 = typedef "Keithley 622x.lvlib/KE6221 -- Wave Playback Num Cycles.ctl" = dbl
  T17 = typedef "Keithley 622x.lvlib/KE6221 -- Wave Phase Marker.ctl" = dbl
  T18 = typedef "Keithley 622x.lvlib/KE622x -- Trig Link Line.ctl" = enum16{"1", "2", "3", "4", "5", "6"}
  T19 = cluster{"Sine Wave Params In":T8, "RMS Amplitude (A)":T10}
  T20 = cluster{"ID Query":bool, "Reset":bool, "Sensitivity 2":i16, "Sensitivity 1":i16, "SR830源配合的阻抗（6221做源可忽略）":dbl, "SR830 2":bool, "SR830 3":bool, "SR830 4":bool, "Sensitivity 3":i16, "Sensitivity 4":i16, "source":u16, "SR830 1":bool, "Reserve 1":i16, "Reserve 2":i16, "Reserve 3":i16, "Reserve 4":i16}
  T21 = cluster{"Time Constant ":u16, "Low Pass Filter Slope ":u16, "Enable Sync Filter ":bool}
  T22 = cluster{"Reference Source":u16, "External Reference Trigger  ":u16, "Detection Harmonic Number ":dbl, "Manual Phase (Degree)":dbl, "Auto Phase ":bool, "Sine Output Amplitude (V)":dbl, "Internal Reference Frequency (Hz)":dbl}
  T23 = cluster{"Input Notch Filter ":u16, "Input Shield Grounding":u16, "Input Coupling ":u16, "Input Connection  ":u16}
  T24 = typedef "Keithley 622x.lvlib/KE6221 -- Wave Type.ctl" = enum16{"Sinusoid", "Square", "Ramp", "Arbitrary 0", "Arbitrary 1", "Arbitrary 2", "Arbitrary 3", "Arbitrary 4"}
  T25 = enum16{"open", "replace", "create", "open or create", "replace or create", "replace or create with confirmation"}
  T26 = typedef "Keithley 622x.lvlib/KE622x -- On Off Control.ctl" = enum16{"Off", "On"}
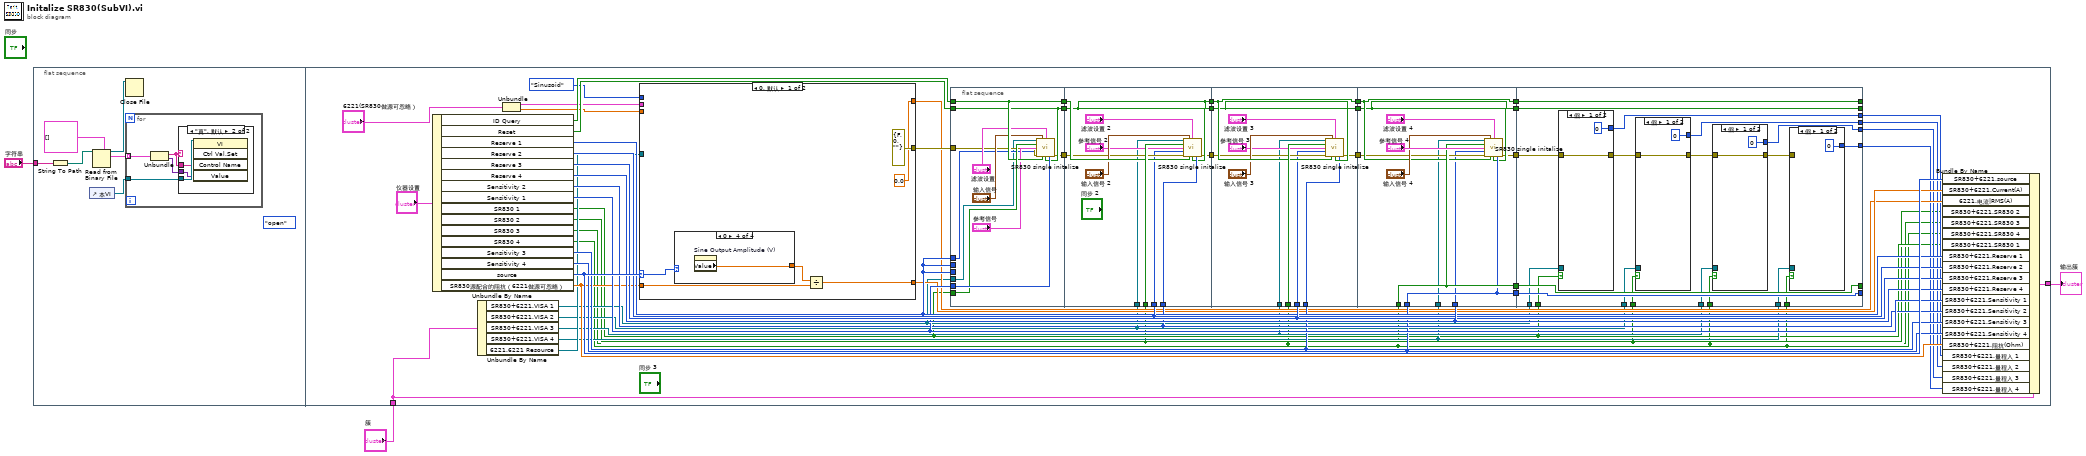
[diagram p0: block diagram]
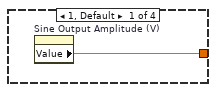
[diagram p3: hidden frame]
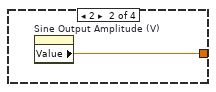
[diagram p4: hidden frame]
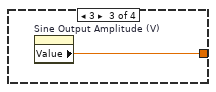
[diagram p5: hidden frame]
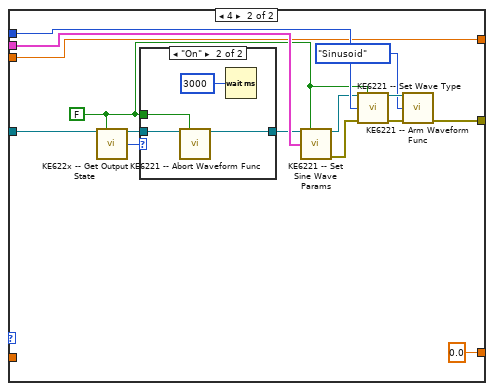
[diagram p6: hidden frame]
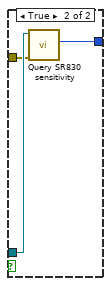
[diagram p8: hidden frame]
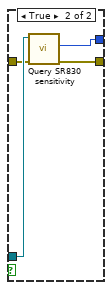
[diagram p9: hidden frame]
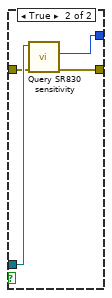
[diagram p10: hidden frame]
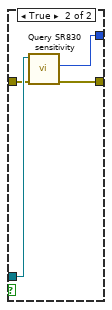
[diagram p11: hidden frame]
diagram:
  n1 = flat-sequence {
    tunnel: "字符串" -> [w4]
    tunnel: "簇" -> [w38]
    tunnel: [w35] -> w1
    frame #0 {
      (unwired) T25."open" ("操作(0:open)")
      n2 = String To Path(string=w4) -> (path=w8:path)
      n3 = control-ref of="本VI"() -> (w9:refnum<vi>)
      n4 = Read from Binary File(5:cluster{"Name":string, "Variant Data":variant}[] [] ("控件值:获取全部"), 11:w8) -> (2:w5:cluster{"Name":string, "Variant Data":variant}[], 3:w7:refnum<file>)  [unwired: 4 in, 2 out]
      n5 = Close File(refnum=w7) -> ()  [unwired: 1 in, 2 out]
      n6 = for {
        tunnel: w5 -> [w13] mode=indexing
        tunnel: w9 -> [w12]
        n7 = Unbundle(w13) -> ("Name"=w10:string, "Variant Data"=w11:variant)
        n8 = case shown="\"真\", 默认" w10 {
          tunnel: w12 -> [_ w16]
          tunnel: w10 -> [_ w15]
          tunnel: w11 -> [_ w14]
          frame "6221", "cancel", "load", "model", "ok" {
          }
          frame "真", Default {
            n9 = invoke class="VI" method="Ctrl Val.Set"(reference=w16, "Control Name"=w15, "Value"=w14) -> ()  [unwired: 2 in, 5 out]
          }
        }
      }
    }
    frame #1 {
      n10 = Unbundle By Name("仪器设置") -> ("ID Query"=w65:bool, "Reset"=w64:bool, "Reserve 1"=w44:i16, "Reserve 2"=w45:i16, "Reserve 3"=w46:i16, "Reserve 4"=w47:i16, "Sensitivity 2"=w42:i16, "Sensitivity 1"=w43:i16, "SR830 1"=w20:bool, "SR830 2"=w19:bool, "SR830 3"=w18:bool, "SR830 4"=w17:bool, "Sensitivity 3"=w41:i16, "Sensitivity 4"=w40:i16, "source"=w52:u16, "SR830源配合的阻抗（6221做源可忽略）"=w39:dbl)
      n11 = Unbundle By Name(w38) -> ("SR830+6221.VISA 1"=w28:refnum<visa-resource-name>, "SR830+6221.VISA 2"=w27:refnum<visa-resource-name>, "SR830+6221.VISA 3"=w26:refnum<visa-resource-name>, "SR830+6221.VISA 4"=w25:refnum<visa-resource-name>, "6221.6221 Resource"=w34:refnum<visa-resource-name>)
      n12 = Unbundle("6221(SR830做源可忽略）") -> ("Sine Wave Params In"=w50:T8, "RMS Amplitude (A)"=w48:T10)
      n13 = case shown="0, 默认" w52 {
        selector: w52 -> [w68 _]
        tunnel: KE6221_--_Wave_Type."Sinusoid" ("Wave Type") -> [_ w90]
        tunnel: [errorcluster {"status"=FALSE, "code"=0, "source"=""} ("error out") w83] -> w53
        tunnel: w50 -> [_ w87]
        tunnel: w34 -> [_ w82]
        tunnel: w48 -> [_ w86]
        tunnel: w39 -> [w69 _]
        tunnel: [T10 0.0 ("RMS Amplitude (A)") w86] -> w36
        tunnel: [w67 0.0] -> w37
        frame 0, Default {
          n14 = case shown="0" w68 {
            tunnel: [w72 w73 w74 w75] -> w70
            frame 1, Default {
              n15 = property on="Sine Output Amplitude (V)" class="DigNum (严格)"() -> ("Value"=w72:dbl)  [unwired: 2 in, 2 out]
            }
            frame 2 {
              n16 = property on="Sine Output Amplitude (V)" class="DigNum (严格)"() -> ("Value"=w73:dbl)  [unwired: 2 in, 2 out]
            }
            frame 3 {
              n17 = property on="Sine Output Amplitude (V)" class="DigNum (严格)"() -> ("Value"=w74:dbl)  [unwired: 2 in, 2 out]
            }
            frame 0 {
              n18 = property on="Sine Output Amplitude (V)" class="DigNum (严格)"() -> ("Value"=w75:dbl)  [unwired: 2 in, 2 out]
            }
          }
          n19 = Divide(x=w70, y=w69) -> (x/y=w67:dbl)
        }
        frame 4 {
          w79 = FALSE ("Check For SCPI Errors? (T)")
          n20 = call "KE622x -- Get Output State.vi"("Resource In"=w82, "Check For SCPI Errors? (T)"=w79) -> ("Resource Out (dupl)"=w80:refnum<visa-resource-name>, "Output State"=w81:T26)  [unwired: 11 in, 1 out]
          n21 = case shown="\"On\"" w81 {
            tunnel: w80 -> [w91 w95]
            tunnel: w79 -> [_ w94]
            tunnel: [w91 w93] -> w78
            frame "Off", Default {
            }
            frame "On" {
              n22 = call "KE6221 -- Abort Waveform Func.vi"("Resource In"=w95, "Check For SCPI Errors? (T)"=w94) -> ("Resource Out (dupl)"=w93:refnum<visa-resource-name>)  [unwired: 12 in, 1 out]
              n23 = Wait (ms)(milliseconds to wait=u32 3000 ("等待时间（毫秒）")) -> ()  [unwired: 1 out]
            }
          }
          n24 = call "KE6221 -- Set Sine Wave Params.vi"("Resource In"=w78, "Check For SCPI Errors? (T)"=w79, "Sine Wave Params In"=w87) -> ("Resource Out (dupl)"=w89:refnum<visa-resource-name>, "error out"=w88:errorcluster)  [unwired: 10 in, 1 out]
          n25 = call "KE6221 -- Set Wave Type.vi"("Resource In"=w89, "Check For SCPI Errors? (T)"=w79, "Wave Type"=w90, "error in (no error)"=w88) -> ("Resource Out (dupl)"=w85:refnum<visa-resource-name>, "error out"=w84:errorcluster)  [unwired: 10 in]
          n26 = call "KE6221 -- Arm Waveform Func.vi"("Resource In"=w85, "Wave Type"=KE6221_--_Wave_Type."Sinusoid", "error in (no error)"=w84) -> ("error out"=w83:errorcluster)  [unwired: 11 in, 1 out]
        }
      }
      n27 = flat-sequence {
        tunnel: w44 -> [_]
        tunnel: w43 -> [w106]
        tunnel: w65 -> [w104]
        tunnel: w64 -> [w103]
        tunnel: w20 -> [w105]
        tunnel: [w104] -> w63
        tunnel: [w103] -> w62
        tunnel: [w99] -> w57
        tunnel: w53 -> [w98]
        tunnel: w44 -> [_]
        tunnel: w44 -> [w97]
        tunnel: w28 -> [w96]
        tunnel: w19 -> [w117]
        tunnel: w42 -> [w116]
        tunnel: w63 -> [w115]
        tunnel: w62 -> [w114]
        tunnel: [w114] -> w61
        tunnel: [w114] -> w60
        tunnel: w57 -> [w110]
        tunnel: [w109] -> w56
        tunnel: w45 -> [w108]
        tunnel: w27 -> [w107]
        tunnel: w18 -> [w128]
        tunnel: w61 -> [w127]
        tunnel: w60 -> [w126]
        tunnel: [w127] -> w59
        tunnel: [w126] -> w58
        tunnel: w56 -> [w122]
        tunnel: [w121] -> w55
        tunnel: w46 -> [w120]
        tunnel: w26 -> [w119]
        tunnel: w41 -> [w118]
        tunnel: w17 -> [w136]
        tunnel: w40 -> [w135]
        tunnel: w59 -> [w134]
        tunnel: w58 -> [w133]
        tunnel: w55 -> [w132]
        tunnel: w47 -> [w130]
        tunnel: w25 -> [w129]
        tunnel: [w136] -> w33
        tunnel: [w133] -> w32
        tunnel: [w134] -> w31
        tunnel: [w135] -> w30
        tunnel: [w131] -> w29
        tunnel: [w156] -> _
        tunnel: [w157] -> _
        tunnel: [w158] -> _
        tunnel: [w159] -> _
        tunnel: w33 -> [w159]
        tunnel: w32 -> [w158]
        tunnel: w31 -> [w157]
        tunnel: w30 -> [w156]
        tunnel: w29 -> [w148]
        tunnel: w28 -> [w155]
        tunnel: w27 -> [w154]
        tunnel: w26 -> [w153]
        tunnel: w25 -> [w152]
        tunnel: [w147] -> w24
        tunnel: [w146] -> w23
        tunnel: [w145] -> w22
        tunnel: [w144] -> w21
        tunnel: w20 -> [w143]
        tunnel: w19 -> [w142]
        tunnel: w18 -> [w141]
        tunnel: w17 -> [w140]
        frame #0 {
          n28 = call "SR830 single initalize.vi"("VISA引用句柄输入"=w96, "输入信号"="输入信号", "滤波设置"="滤波设置", "open"=w105, "参考信号"="参考信号", "Reserve"=w97, "error in (no error)"=w98, "ID Query (True)"=w104, "Reset (True)"=w103, "Sensitivity (-1: Auto gain)"=w106) -> ("错误输出"=w99:cluster{"status":bool, "code":i32, string})  [unwired: 5 in]
        }
        frame #1 {
          n29 = call "SR830 single initalize.vi"("VISA引用句柄输入"=w107, "输入信号"="输入信号 2", "滤波设置"="滤波设置 2", "open"=w117, "参考信号"="参考信号 2", "Reserve"=w108, "error in (no error)"=w110, "ID Query (True)"=w115, "Reset (True)"=w114, "Sensitivity (-1: Auto gain)"=w116) -> ("错误输出"=w109:cluster{"status":bool, "code":i32, string})  [unwired: 5 in]
        }
        frame #2 {
          n30 = call "SR830 single initalize.vi"("VISA引用句柄输入"=w119, "输入信号"="输入信号 3", "滤波设置"="滤波设置 3", "open"=w128, "参考信号"="参考信号 3", "Reserve"=w120, "error in (no error)"=w122, "ID Query (True)"=w127, "Reset (True)"=w126, "Sensitivity (-1: Auto gain)"=w118) -> ("错误输出"=w121:cluster{"status":bool, "code":i32, string})  [unwired: 5 in]
        }
        frame #3 {
          n31 = call "SR830 single initalize.vi"("VISA引用句柄输入"=w129, "输入信号"="输入信号 4", "滤波设置"="滤波设置 4", "open"=w136, "参考信号"="参考信号 4", "Reserve"=w130, "error in (no error)"=w132, "ID Query (True)"=w134, "Reset (True)"=w133, "Sensitivity (-1: Auto gain)"=w135) -> ("错误输出"=w131:cluster{"status":bool, "code":i32, string})  [unwired: 5 in]
        }
        frame #4 {
          n32 = case shown="假" w143 {
            tunnel: w155 -> [_ w181]
            tunnel: [w176 w180] -> w149
            tunnel: w148 -> [w176 w179]
            tunnel: [0 ("sensitivity") w178] -> w147
            frame False {
            }
            frame True {
              n33 = call "Query SR830 sensitivity.vi"("error in (no error)"=w179, "VISA resource name"=w181) -> ("错误输出"=w180:errorcluster, "sensitivity"=w178:i32)  [unwired: 7 in, 1 out]
            }
          }
          n34 = case shown="假" w142 {
            tunnel: w154 -> [_ w175]
            tunnel: [w171 w174] -> w150
            tunnel: w149 -> [w171 w173]
            tunnel: [0 ("sensitivity") w172] -> w146
            frame False {
            }
            frame True {
              n35 = call "Query SR830 sensitivity.vi"("error in (no error)"=w173, "VISA resource name"=w175) -> ("错误输出"=w174:errorcluster, "sensitivity"=w172:i32)  [unwired: 7 in, 1 out]
            }
          }
          n36 = case shown="假" w141 {
            tunnel: w153 -> [_ w169]
            tunnel: [w164 w168] -> w151
            tunnel: w150 -> [w164 w167]
            tunnel: [0 ("sensitivity") w166] -> w145
            frame False {
            }
            frame True {
              n37 = call "Query SR830 sensitivity.vi"("error in (no error)"=w167, "VISA resource name"=w169) -> ("错误输出"=w168:errorcluster, "sensitivity"=w166:i32)  [unwired: 7 in, 1 out]
            }
          }
          n38 = case shown="假" w140 {
            tunnel: w152 -> [_ w163]
            tunnel: w151 -> [_ w162]
            tunnel: [0 ("sensitivity") w161] -> w144
            frame False {
            }
            frame True {
              n39 = call "Query SR830 sensitivity.vi"("error in (no error)"=w162, "VISA resource name"=w163) -> ("sensitivity"=w161:i32)  [unwired: 7 in, 2 out]
            }
          }
        }
      }
      n40 = Bundle By Name(cluster=w38, "SR830+6221.source"=w52, "SR830+6221.Current(A)"=w37, "6221.电流|RMS(A)"=w36, "SR830+6221.SR830 2"=w19, "SR830+6221.SR830 3"=w18, "SR830+6221.SR830 4"=w17, "SR830+6221.SR830 1"=w20, "SR830+6221.Reserve 1"=w44, "SR830+6221.Reserve 2"=w45, "SR830+6221.Reserve 3"=w46, "SR830+6221.Reserve 4"=w47, "SR830+6221.Sensitivity 1"=w43, "SR830+6221.Sensitivity 2"=w42, "SR830+6221.Sensitivity 3"=w41, "SR830+6221.Sensitivity 4"=w40, "SR830+6221.阻抗(Ohm)"=w39, "SR830+6221.量程入 1"=w24, "SR830+6221.量程入 2"=w23, "SR830+6221.量程入 3"=w22, "SR830+6221.量程入 4"=w21) -> (w35:T1)
    }
  }
  "输出簇" <- w1
